vi "ReadSizeMat_1DArray-U32_Color.vi"(8 "error in":errorcluster, 11 "Array in":u32[](array[numeric])) -> (0 "error out":errorcluster, 1 "Height":i32, 2 "Width":i32, 3 "Array out":u32[](array[numeric]), 4 "Channel":i32)   [LabVIEW 2020, in "OpenLvVision_OpenCv.lvlib"]
doc: "Read size of the datatype\nNo malleable to breake vi inlining!"
uses:
  OpenLvVision_OpenCv.lvlib
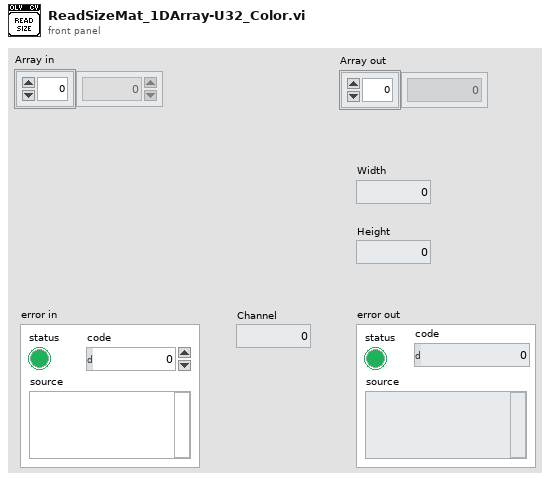
[diagram p1: front panel]
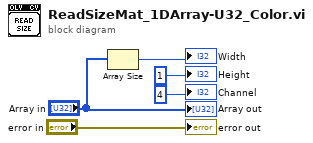
[diagram p0: block diagram]
diagram:
  n1 = Array Size(array="Array in") -> (size(s)=→"Width":i32)
  "error out" <- "error in"
  "Height" <- 1
  "Channel" <- 4
  "Array out" <- "Array in"
